vi "Disabled.vi"(7 "Robot Mode":T2, 10 "Match Info":T1={"Autonomous Elapsed Seconds"=0.0, "TeleOp Elapsed Seconds"=0.0, "Disabled Elapsed Seconds"=0.0, "Visited Autonomous"=FALSE, "Visited TeleOp"=FALSE, "Visited Disabled"=FALSE, "Autonomous Settings"={"Autonomous Style"=enum."Independent", "VI Refnum"=refnum}}, 11 "Call Context":T3) -> ()   [LabVIEW 2011]
doc: "This VI is called each time a disabled packet is received from the DS. It is often used to prepare for the next robot mode, to calibrate sensors, etc."
uses:
  <vilib>/Rock Robotics/WPI/DriverStation/WPI_DriverStationDerivedRobotMode.ctl
  <vilib>/Rock Robotics/WPI/DriverStation/WPI_DriverStationRobotMode.ctl
  <vilib>/Rock Robotics/WPI/DriverStation/WPI_DriverStationMatch Info.ctl
  <vilib>/Rock Robotics/WPI/DriverStation/DriverStationLCD/WPI_DriverStationLCDLCDLine.ctl
  GLOBALShooter.vi
  GLOBALBridge.vi
  GLOBALHarvester.vi
  GLOBALDriveTrain.vi
  GLOBALMain.vi
  <vilib>/Utility/file.llb/Read From Spreadsheet File (DBL).vi
panel:
  out "Path and file":string
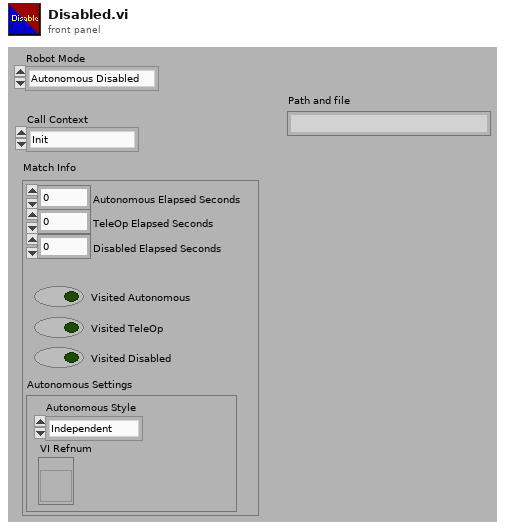
[diagram p1: front panel]
types:
  T1 = typedef "WPI_DriverStationMatch Info.ctl" = cluster{"Autonomous Elapsed Seconds":dbl, "TeleOp Elapsed Seconds":dbl, "Disabled Elapsed Seconds":dbl, "Visited Autonomous":bool, "Visited TeleOp":bool, "Visited Disabled":bool, "Autonomous Settings":cluster{"Autonomous Style":enum16{"Iterative", "Independent"}, "VI Refnum":refnum<vi>}}
  T2 = typedef "WPI_DriverStationRobotMode.ctl" = enum16{"Autonomous Disabled", "Autonomous Enabled", "Teleop Disabled", "Teleop Enabled", "Timeout", "Finish"}
  T3 = typedef "WPI_DriverStationDerivedRobotMode.ctl" = enum16{"Init", "Execute", "Stop"}
  T4 = typedef "WPI_DriverStationLCDLCDLine.ctl" = enum16{"Main - Line 1", "User - Line 2", "User - Line 3", "User - Line 4", "User - Line 5", "User - Line 6"}
  T5 = typedef "WPI_JoystickDevRef.ctl" = cluster{"Device":T6}
  T6 = typedef "WPI_JoystickDeviceEnum.ctl" = enum16{"USB 1", "USB 2", "USB 3", "USB 4", "Kinect 1", "Kinect 2"}
  T7 = cluster{"Shifting":cluster{"Right Servo High":dbl, "Right Servo Low":dbl, "Left Servo High":dbl, "Left Servo Low":dbl}, "Breaking":cluster{"Coast Position":dbl, "Break Position":dbl}}
  T8 = typedef "WPI_JoystickButtonState.ctl" = cluster{"Button 1":bool, "Button 2":bool, "Button 3":bool, "Button 4":bool, "Button 5":bool, "Button 6":bool, "Button 7":bool, "Button 8":bool, "Button 9":bool, "Button 10":bool, "Button 11":bool, "Button 12":bool}
  T9 = cluster{"Right Servo High":dbl, "Right Servo Low":dbl, "Left Servo High":dbl, "Left Servo Low":dbl}
  T10 = cluster{"Coast Position":dbl, "Break Position":dbl}
  T11 = typedef "WPI_ServoDeviceRef.ctl" = cluster{"DeviceStatus":errorcluster, "Digital Module":T12, "PWM Channel":T13, "DeadBand":T14}
  T12 = typedef "FPGA_TypedefDigitalModule.ctl" = enum16{"Digital Module 1", "Digital Module 2"}
  T13 = typedef "FPGA_DIOPWMChannel.ctl" = enum8{"PWM 1", "PWM 2", "PWM 3", "PWM 4", "PWM 5", "PWM 6", "PWM 7", "PWM 8", "PWM 9", "PWM 10", "Invalid"}
  T14 = typedef "WPI_PWMDeadband.ctl" = cluster{"Name":string, "maxPositivePwm":i32, "minPositivePwm":i32, "centerPwm":i32, "maxNegativePwm":i32, "minNegativePwm":i32, "angularRange":u16}
  T15 = typedef "WPI_MotorControlDeviceRef.ctl" = cluster{"DeviceStatus":errorcluster, "Type":enum16{"PWM", "CAN"}, "PWM":cluster{"Digital Module":T12, "PWM Channel":T13, "DeadBand":T14}, "CAN":cluster{"Device Number":u8, "Control Mode":T16, "Semaphore":T17, "Max Vout":dbl}, "Invert":bool, "TransformRef":T18, "InvTransformRef":T18}
  T16 = typedef "WPI_CANJaguar_ControlMode.ctl" = enum8{"Percent VBus", "Current", "Speed", "Position", "Voltage"}
  T17 = typedef "Semaphore RefNum" = refnum<k1>
  T18 = typedef "WPI_PWMTransform_ConPane.ctl" = refnum<vi>
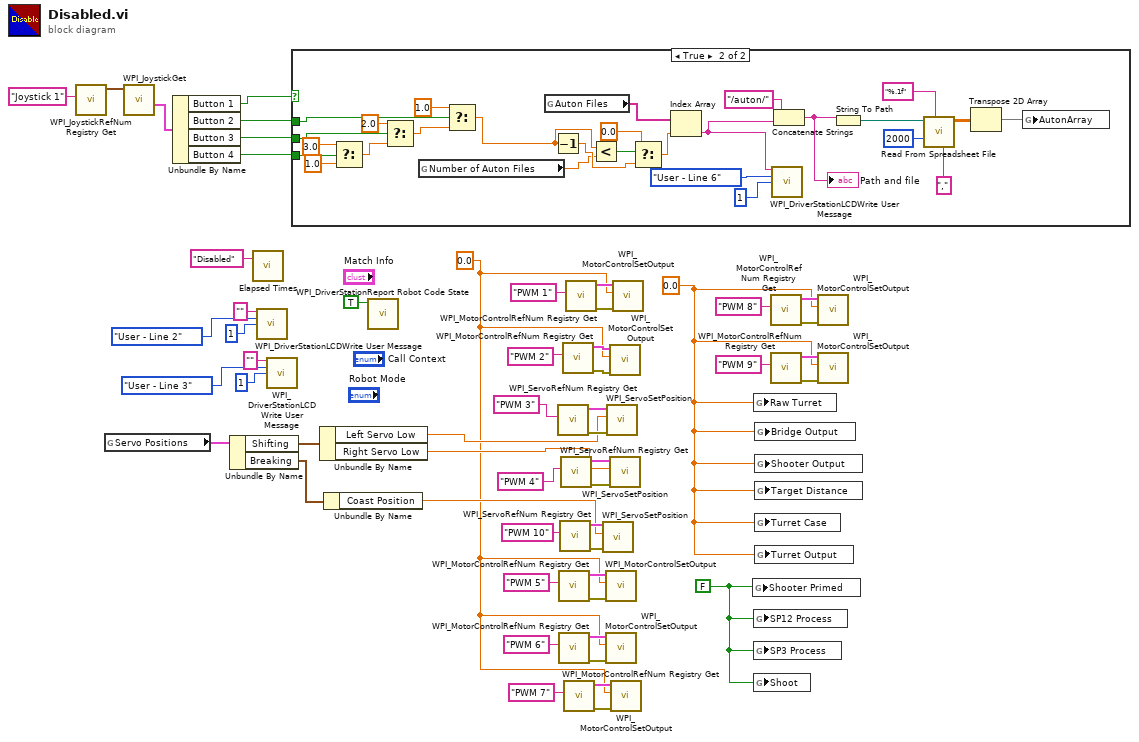
[diagram p0: block diagram]
diagram:
  w2 = FALSE ("Shooter Primed")
  w3 = 0.0 ("Raw Turret")
  w4 = 0.0 ("Raw Turret")
  n1 = call <vilib>:"WPI_JoystickRefNum Registry Get.vi"("refnum name"="Joystick 1") -> ("JoystickDevRef"=w31:T5)  [unwired: 9 in, 1 out]
  n2 = global read "GLOBALDriveTrain.vi" "Servo Positions"() -> (w16:T7)
  n3 = call <vilib>:"WPI_JoystickGet.vi"("JoystickDevRef"=w31) -> ("Buttons"=w30:T8)  [unwired: 4 in, 2 out]
  n4 = Unbundle By Name(w30) -> ("Button 1"=w29:bool, "Button 2"=w28:bool, "Button 3"=w27:bool, "Button 4"=w26:bool)
  n5 = Unbundle By Name(w16) -> ("Shifting"=w15:T9, "Breaking"=w6:T10)
  n6 = call "Elapsed Times.vi"("Call Name"="Disabled") -> ()  [unwired: 2 in, 1 out]
  n7 = call <vilib>:"WPI_DriverStationLCDWrite User Message.vi"("line text"="", "line"=WPI_DriverStationLCDLCDLine."User - Line 2", "starting column"=i8 1) -> ()  [unwired: 2 in, 11 out]
  n8 = call <vilib>:"WPI_DriverStationLCDWrite User Message.vi"("line text"="", "line"=WPI_DriverStationLCDLCDLine."User - Line 3", "starting column"=i8 1) -> ()  [unwired: 2 in, 11 out]
  n9 = case shown="True" w29 {
    tunnel: w28 -> [_ w78]
    tunnel: w27 -> [_ w76]
    tunnel: w26 -> [_ w81]
    frame False {
    }
    frame True {
      n10 = Select(t=3.0, s=w81, f=1.0) -> (s? t:f=w74:dbl)
      n11 = Select(t=2.0, s=w76, f=w74) -> (s? t:f=w73:dbl)
      n12 = global read "GLOBALMain.vi" "Number of Auton Files"() -> (w65:dbl)
      n13 = Select(t=1.0, s=w78, f=w73) -> (s? t:f=w66:dbl)
      n14 = global read "GLOBALMain.vi" "Auton Files"() -> (w64:string[])
      n15 = Decrement(x=w66) -> (x-1=w67:dbl)
      n16 = Less?(x=w66, y=w65) -> (x < y?=w70:bool)
      n17 = Select(t=0.0, s=w70, f=w67) -> (s? t:f=w68:dbl)
      n18 = Index Array(array=w64, index=w68) -> (element=w56:string)
      n19 = call <vilib>:"WPI_DriverStationLCDWrite User Message.vi"("line text"=w56, "line"=WPI_DriverStationLCDLCDLine."User - Line 6", "starting column"=i8 1) -> ()  [unwired: 2 in, 11 out]
      n20 = Concatenate Strings("/auton/" ("string"), w56) -> (w60:string)
      "Path and file" <- w60
      n21 = String To Path(string=w60) -> (path=w61:path)
      n22 = call-poly <vilib>:"Read From Spreadsheet File.vi"("delimiter (\\t)"="," ("delimiter (\\t)"), "format (%.3f)"="%.1f", "number of rows (all:-1)"=2000, "file path (dialog if empty)"=w61) -> ("all rows"=w55:dbl[][])  [unwired: 1 in, 6 out]
      n23 = Transpose 2D Array(2D array=w55) -> (transposed array=w63:dbl[][])
      n24 = global write "GLOBALMain.vi" "AutonArray"(w63) -> ()
    }
  }
  n25 = Unbundle By Name(w15) -> ("Left Servo Low"=w11:dbl, "Right Servo Low"=w10:dbl)
  n26 = Unbundle By Name(w6) -> ("Coast Position"=w5:dbl)
  n27 = call <vilib>:"WPI_DriverStationReport Robot Code State.vi"("Disabled"=TRUE ("Autonomous")) -> ()  [unwired: 10 in, 1 out]
  n28 = call <vilib>:"WPI_ServoRefNum Registry Get.vi"("refnum name"="PWM 3") -> ("error out"=w14:errorcluster, "ServoDeviceRef"=w13:T11)  [unwired: 9 in]
  n29 = call <vilib>:"WPI_MotorControlRefNum Registry Get.vi"("refnum name"="PWM 5") -> ("error out"=w46:errorcluster, "MotorControlDevRef"=w47:T15)  [unwired: 9 in]
  n30 = call <vilib>:"WPI_MotorControlRefNum Registry Get.vi"("refnum name"="PWM 6") -> ("error out"=w43:errorcluster, "MotorControlDevRef"=w42:T15)  [unwired: 9 in]
  n31 = call <vilib>:"WPI_ServoRefNum Registry Get.vi"("refnum name"="PWM 10") -> ("error out"=w19:errorcluster, "ServoDeviceRef"=w18:T11)  [unwired: 9 in]
  n32 = call <vilib>:"WPI_ServoRefNum Registry Get.vi"("refnum name"="PWM 4") -> ("error out"=w12:errorcluster, "ServoDeviceRef"=w9:T11)  [unwired: 9 in]
  n33 = call <vilib>:"WPI_MotorControlRefNum Registry Get.vi"("refnum name"="PWM 2") -> ("error out"=w49:errorcluster, "MotorControlDevRef"=w48:T15)  [unwired: 9 in]
  n34 = call <vilib>:"WPI_MotorControlRefNum Registry Get.vi"("refnum name"="PWM 7") -> ("error out"=w40:errorcluster, "MotorControlDevRef"=w41:T15)  [unwired: 9 in]
  n35 = call <vilib>:"WPI_MotorControlRefNum Registry Get.vi"("refnum name"="PWM 1") -> ("error out"=w52:errorcluster, "MotorControlDevRef"=w53:T15)  [unwired: 9 in]
  n36 = call <vilib>:"WPI_ServoSetPosition.vi"("error in (no error)"=w19, "Position"=w5, "ServoDeviceRef"=w18) -> ()  [unwired: 7 in, 2 out]
  n37 = call <vilib>:"WPI_MotorControlSetOutput.vi"("error in (no error)"=w46, "Output"=w3, "MotorControlDevRef"=w47) -> ()  [unwired: 7 in, 2 out]
  n38 = call <vilib>:"WPI_MotorControlSetOutput.vi"("error in (no error)"=w43, "Output"=w3, "MotorControlDevRef"=w42) -> ()  [unwired: 7 in, 2 out]
  n39 = call <vilib>:"WPI_ServoSetPosition.vi"("error in (no error)"=w14, "Position"=w11, "ServoDeviceRef"=w13) -> ()  [unwired: 7 in, 2 out]
  n40 = call <vilib>:"WPI_MotorControlSetOutput.vi"("error in (no error)"=w49, "Output"=w3, "MotorControlDevRef"=w48) -> ()  [unwired: 7 in, 2 out]
  n41 = call <vilib>:"WPI_ServoSetPosition.vi"("error in (no error)"=w12, "Position"=w10, "ServoDeviceRef"=w9) -> ()  [unwired: 7 in, 2 out]
  n42 = call <vilib>:"WPI_MotorControlSetOutput.vi"("error in (no error)"=w40, "Output"=w3, "MotorControlDevRef"=w41) -> ()  [unwired: 7 in, 2 out]
  n43 = call <vilib>:"WPI_MotorControlSetOutput.vi"("error in (no error)"=w52, "Output"=w3, "MotorControlDevRef"=w53) -> ()  [unwired: 7 in, 2 out]
  n44 = global write "GLOBALShooter.vi" "Shooter Primed"(w2) -> ()
  n45 = global write "GLOBALShooter.vi" "Raw Turret"(w4) -> ()
  n46 = global write "GLOBALHarvester.vi" "SP12 Process"(w2) -> ()
  n47 = global write "GLOBALHarvester.vi" "SP3 Process"(w2) -> ()
  n48 = global write "GLOBALHarvester.vi" "Shoot"(w2) -> ()
  n49 = global write "GLOBALBridge.vi" "Bridge Output"(w4) -> ()
  n50 = global write "GLOBALShooter.vi" "Shooter Output"(w4) -> ()
  n51 = global write "GLOBALShooter.vi" "Target Distance"(w4) -> ()
  n52 = global write "GLOBALShooter.vi" "Turret Case"(w4) -> ()
  n53 = global write "GLOBALShooter.vi" "Turret Output"(w4) -> ()
  n54 = call <vilib>:"WPI_MotorControlRefNum Registry Get.vi"("refnum name"="PWM 8") -> ("error out"=w37:errorcluster, "MotorControlDevRef"=w36:T15)  [unwired: 9 in]
  n55 = call <vilib>:"WPI_MotorControlRefNum Registry Get.vi"("refnum name"="PWM 9") -> ("error out"=w34:errorcluster, "MotorControlDevRef"=w35:T15)  [unwired: 9 in]
  n56 = call <vilib>:"WPI_MotorControlSetOutput.vi"("error in (no error)"=w37, "Output"=w4, "MotorControlDevRef"=w36) -> ()  [unwired: 7 in, 2 out]
  n57 = call <vilib>:"WPI_MotorControlSetOutput.vi"("error in (no error)"=w34, "Output"=w4, "MotorControlDevRef"=w35) -> ()  [unwired: 7 in, 2 out]
